vi "CAL-Smooth.vi"(1 "Magnitude":dbl[](array[numeric])) -> (0 "Magnitude Smoothed":dbl[](array[numeric]))   [LabVIEW 2020]
uses:
  <vilib>/Analysis/3filter.llb/Savitzky-Golay Filter (DBL).vi
  <vilib>/Analysis/NI_AALBase.lvlib
panel:
  out "error":i32
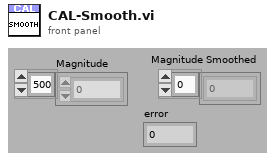
[diagram p1: front panel]
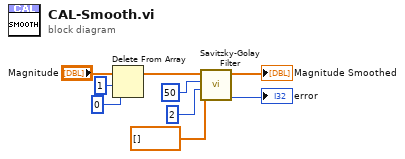
[diagram p0: block diagram]
diagram:
  n1 = Delete From Array(array="Magnitude", length=1, index=0) -> (array with subset deleted=w6:dbl[])  [unwired: 1 out]
  n2 = call-poly <vilib>:"Savitzky-Golay Filter.vi"("Weight"=dbl[] [], "polynomial order"=2, "side points"=50, "X"=w6) -> ("error"=→"error":i32, "Filtered X"=→"Magnitude Smoothed":dbl[])  [unwired: 6 in]
